vi "binary search3VIwithRenormalization.vi"(6 "Renormalization Factor":sgl, 7 "Rg2":sgl, 8 "X0":sgl=0.5, 9 "right domain":sgl=18.0, 11 "array":sgl[](array[numeric])) -> (0 "size(s)":i32=1024, 1 "Xmin":sgl, 2 "Xmax":sgl, 3 "Xpot":sgl, 5 "dx":sgl)   [LabVIEW 2019]
panel:
  out "Actual index":sgl=296.33334
  out "right":i32=297
  out "left/index":i32=296
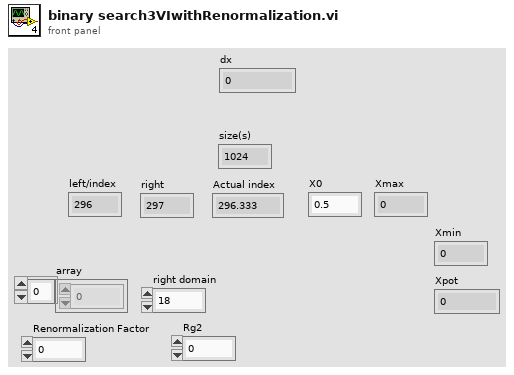
[diagram p1: front panel]
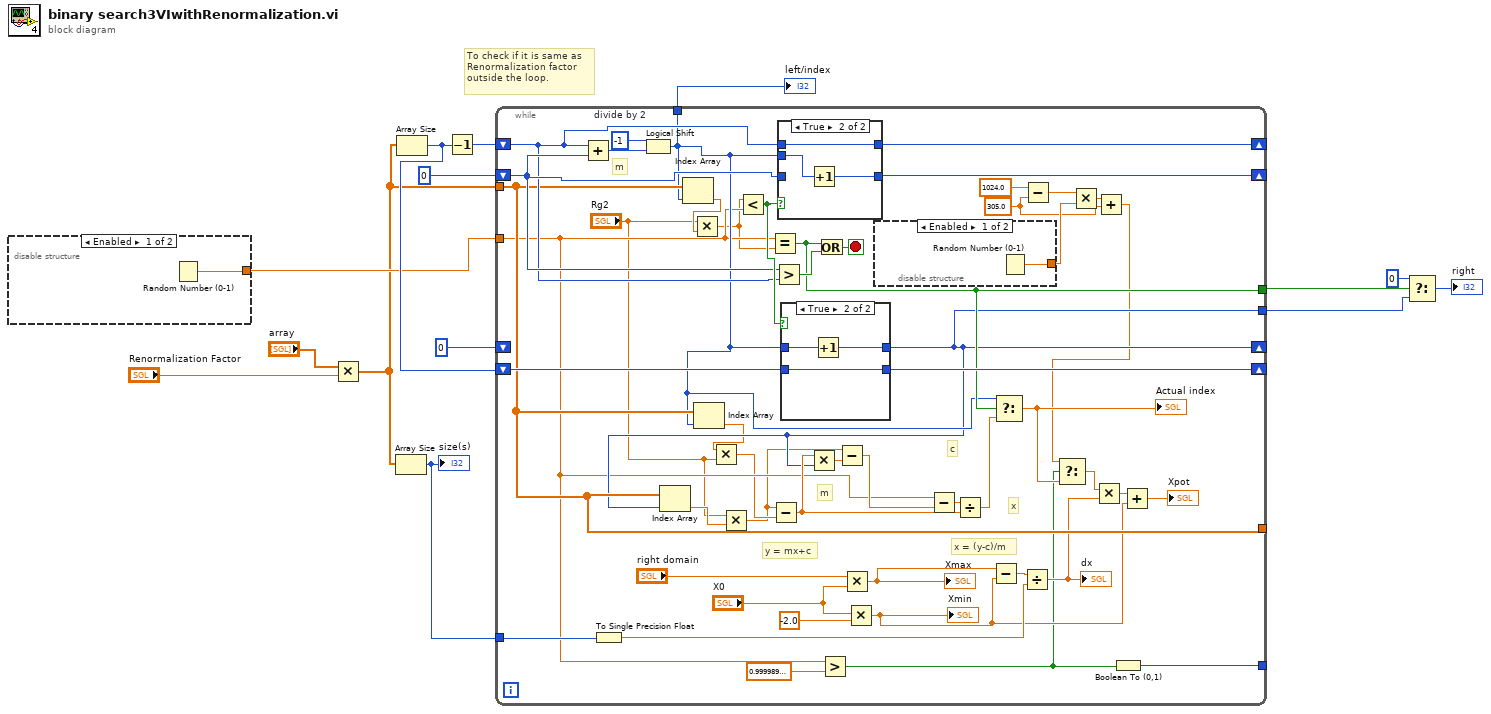
[diagram p0: block diagram]
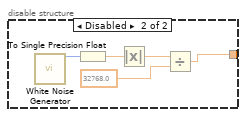
[diagram p2: hidden frame]
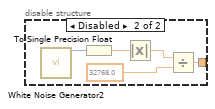
[diagram p3: hidden frame]
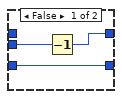
[diagram p5: hidden frame]
diagram:
  # "To check if it is same as \nRenormalization factor\noutside the loop."
  n1 = disable-structure shown="Enabled" {
    disable-tunnel: [w15 w16] -> w4
    frame Enabled {
      n2 = Random Number (0-1)() -> (number: 0 to 1=w15:dbl)
    }
    frame Disabled {
      n3 = call "White Noise Generator"() -> ("white noise out"=w20:i16)  [unwired: 15 in]
      n4 = To Single Precision Float(number=w20) -> (single precision float=w18:sgl)
      n5 = Absolute Value(x=w18) -> (abs(x)=w17:sgl)
      n6 = Divide(x=w17, y=sgl 32768.0) -> (x/y=w16:sgl)
    }
  }
  n7 = Multiply(x="array", y="Renormalization Factor") -> (x*y=w1:sgl[])
  n8 = Array Size(array=w1) -> (size(s)=w5:i32)
  "size(s)" <- w5
  n9 = Array Size(array=w1) -> (size(s)=w7:i32)
  n10 = Decrement(x=w7) -> (x-1=w8:i32)
  n11 = while {
    tunnel: w1 -> [w59]
    tunnel: w4 -> [w40]
    shift-right: [w69] -> _
    shift-left: w8 -> [w60]
    shift-right: [w65] -> _
    shift-left: 0 -> [w61]
    shift-right: [w51] -> _
    shift-left: 0 -> [_]
    shift-right: [w62] -> _
    shift-left: w7 -> [w63]
    tunnel: [w57] -> w6
    tunnel: [w51] -> w13
    tunnel: [w58] -> w14
    tunnel: [w59] -> _
    tunnel: w5 -> [w46]
    tunnel: [w29] -> _
    stop <- w67 stop-if-true
    w33 = sgl 305.0 ("y")
    w70 = -1  # divide by 2
    # "x"
    # "x = (y-c)/m"
    # "c"
    # "m"
    # "y = mx+c"
    # "m"
    n12 = Add(x=w60, y=w61) -> (x+y=w66:i32)
    n13 = To Single Precision Float(number=w46) -> (single precision float=w45:sgl)
    n14 = Logical Shift(y=w70, x=w66) -> (x << y=w57:i32)
    n15 = Index Array(array=w59, index=w57) -> (element=w27:sgl)
    n16 = Multiply(x="Rg2", y=w27) -> (x*y=w26:sgl)
    n17 = Index Array(array=w59, index=w57) -> (element=w25:sgl)
    n18 = Multiply(x=w25, y="Rg2") -> (x*y=w24:sgl)
    n19 = Less?(x=w26, y=w40) -> (x < y?=w64:bool)
    n20 = Equal?(x=w40, y=w26) -> (x = y?=w58:bool)
    n21 = Greater?(x=w61, y=w60) -> (0:w68:bool)
    n22 = case shown="True" w64 {
      tunnel: w57 -> [w84 w87]
      tunnel: [w83 w85] -> w69
      tunnel: w61 -> [w82 _]
      tunnel: [w82 w86] -> w65
      tunnel: w60 -> [_ w85]
      frame False {
        n23 = Decrement(x=w84) -> (x-1=w83:i32)
      }
      frame True {
        n24 = Increment(x=w87) -> (x+1=w86:i32)
      }
    }
    n25 = case shown="True" w64 {
      tunnel: w57 -> [w78 w81]
      tunnel: [w77 w80] -> w51
      tunnel: w63 -> [w77 w79]
      tunnel: [w78 w79] -> w62
      frame False {
      }
      frame True {
        n26 = Increment(x=w81) -> (x+1=w80:i32)
      }
    }
    n27 = Index Array(array=w59, index=w51) -> (element=w23:sgl)
    n28 = Multiply(x="Rg2", y=w23) -> (x*y=w21:sgl)
    n29 = Subtract(x=w21, y=w24) -> (x-y=w53:sgl)
    n30 = Multiply(x=w53, y=w51) -> (x*y=w56:sgl)
    n31 = Or(x=w58, y=w68) -> (x .or. y?=w67:bool)
    n32 = Greater?(x=w40, y=sgl 0.99999) -> (0:w30:bool)
    n33 = Subtract(x=w21, y=w56) -> (x-y=w55:sgl)
    n34 = Multiply(x="right domain", y="X0") -> (x*y=w49:sgl)
    "Xmax" <- w49
    n35 = Multiply(x="X0", y=sgl -2.0) -> (x*y=w43:sgl)
    "Xmin" <- w43
    n36 = disable-structure shown="Enabled" {
      disable-tunnel: [w71 w72] -> w35
      frame Enabled {
        n37 = Random Number (0-1)() -> (number: 0 to 1=w71:dbl)
      }
      frame Disabled {
        n38 = call "White Noise Generator2"() -> ("white noise out"=w76:i16)  [unwired: 15 in]
        n39 = To Single Precision Float(number=w76) -> (single precision float=w74:sgl)
        n40 = Absolute Value(x=w74) -> (abs(x)=w73:sgl)
        n41 = Divide(x=w73, y=sgl 32768.0) -> (x/y=w72:sgl)
      }
    }
    n42 = Subtract(x=w40, y=w55) -> (x-y=w54:dbl)
    n43 = Divide(x=w54, y=w53) -> (x/y=w52:dbl)
    n44 = Subtract(x=w49, y=w43) -> (x-y=w48:sgl)
    n45 = Select(t=w57, s=w58, f=w52) -> (s? t:f=w38:dbl)
    "Actual index" <- w38
    n46 = Divide(x=w48, y=w45) -> (x/y=w47:sgl)
    "dx" <- w47
    n47 = Subtract(x=sgl 1024.0, y=w33) -> (x-y=w36:sgl)
    n48 = Multiply(x=w36, y=w35) -> (x*y=w34:dbl)
    n49 = Add(x=w34, y=w33) -> (x+y=w31:dbl)
    n50 = Select(t=w31, s=w30, f=w38) -> (s? t:f=w32:dbl)
    n51 = Multiply(x=w32, y=w47) -> (x*y=w44:dbl)
    n52 = Boolean To (0,1)(Boolean=w30) -> (0, 1=w29:i16)
    n53 = Add(x=w44, y=w43) -> (x+y=→"Xpot":dbl)
  }
  "left/index" <- w6
  n54 = Select(t=0, s=w14, f=w13) -> (s? t:f=→"right":i32)
